vi "Start Module with Retry.vi"(11 "Cfg File Path":path) -> (0 "error out":errorcluster, 1 "Wait for Event Sync?":bool, 2 "Tool Module Broadcast Events":T1)   [LabVIEW 2015, in "Tool Module.lvlib"]
uses:
  Tool Module.lvlib
  Broadcast Events--cluster.ctl
  Did Init Argument--cluster.ctl
  Status Updated Argument--cluster.ctl
  Error Reported Argument--cluster.ctl
  Stop Argument--cluster.ctl
  Get Module Execution Status Argument--cluster.ctl
  Send Status Argument--cluster.ctl
  _STATUS Typedef--cluster.ctl
  Trigger Argument--cluster.ctl
  Connected Argument--cluster.ctl
  Read from File Rtn Argument--cluster.ctl
  Device Temperature Argument--cluster.ctl
  Tool Typedefs/_Temperature All Arrays--typedef.ctl
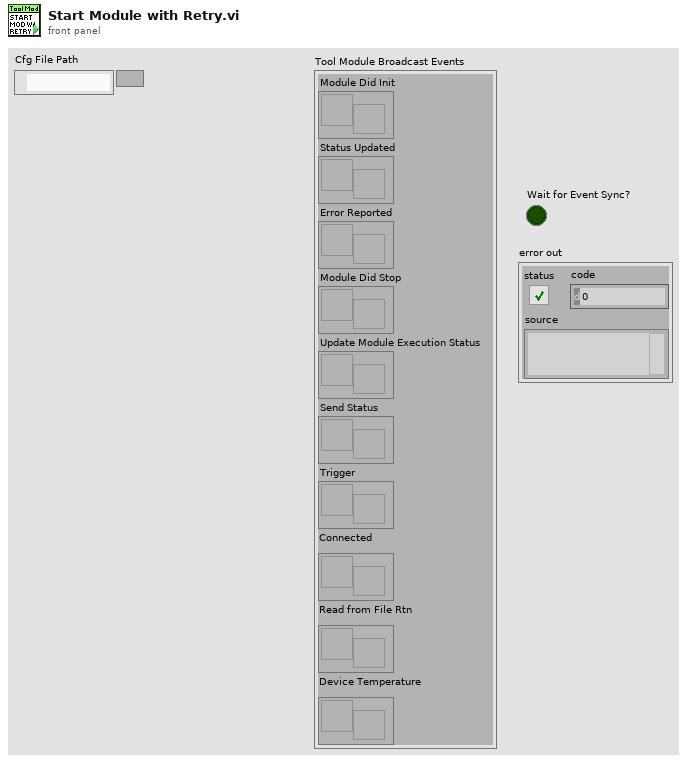
[diagram p1: front panel]
types:
  T1 = typedef "Tool Module.lvlib/Broadcast Events--cluster.ctl" = cluster{"Module Did Init":refnum<user-event>, "Status Updated":refnum<user-event>, "Error Reported":refnum<user-event>, "Module Did Stop":refnum<user-event>, "Update Module Execution Status":refnum<user-event>, "Send Status":refnum<user-event>, "Trigger":refnum<user-event>, "Connected":refnum<user-event>, "Read from File Rtn":refnum<user-event>, "Device Temperature":refnum<user-event>}
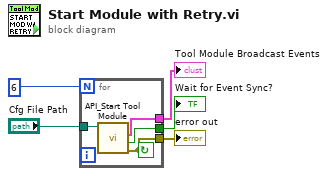
[diagram p0: block diagram]
diagram:
  n1 = for {
    N: 6 -> [_]
    tunnel: "Cfg File Path" -> [w9]
    tunnel: [w6] -> w4
    tunnel: [w8] -> w3
    tunnel: [w7] -> w2
    stop <- w6 continue-if-true
    n2 = call "API_Start Tool Module.vi"("Cfg File Path"=w9) -> ("error out"=w6:errorcluster, "Wait for Event Sync?"=w8:bool, "Tool Module Broadcast Events"=w7:T1)  [unwired: 8 in]
  }
  "error out" <- w4
  "Wait for Event Sync?" <- w3
  "Tool Module Broadcast Events" <- w2
